vi "task01.vi"() -> ()   [LabVIEW 2021]
panel:
  in  "deley":dbl(knob) scale=0.0..2000.0
  out "Waveform Chart":dbl(graph)=0.655447517935951
  out "Numeric":dbl
  in  "Boolean":bool
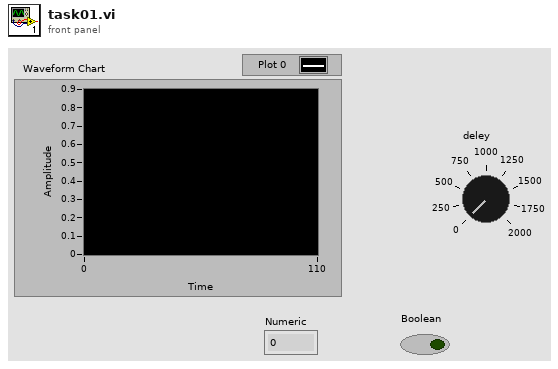
[diagram p1: front panel]
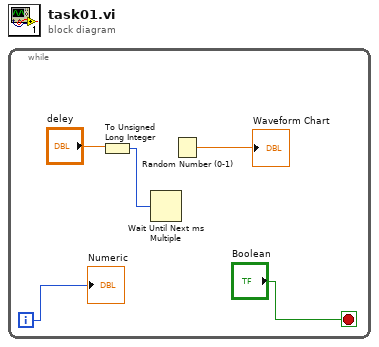
[diagram p0: block diagram]
diagram:
  n1 = while {
    i -> [w4]
    stop <- "Boolean" stop-if-true
    n2 = To Unsigned Long Integer(number="deley") -> (unsigned 32bit integer=w1:u32)
    n3 = Wait Until Next ms Multiple(millisecond multiple=w1) -> ()  [unwired: 1 out]
    n4 = Random Number (0-1)() -> (number: 0 to 1=→"Waveform Chart":dbl)
    "Numeric" <- w4
  }
